vi "Beam deflector.vi"(6 "Sweep direction":bool, 7 "Level #":u8, 8 "Imbalance (V)":dbl min=-10.0 max=10.0 step=0.1 format="%.3f", 9 "Position (V)":dbl min=-10.0 max=10.0 step=0.1 format="%.3g", 10 "Angle (V)":dbl min=-10.0 max=10.0 step=0.1 format="%.3g", 11 "Focus (V)":dbl min=-10.0 max=10.0 step=0.1 format="%.3g") -> (3 "All posts":dbl[][](graph))   [LabVIEW 2018]
uses:
  <vilib>/Analysis/1siggen.llb/Ramp Pattern by Samples.vi
  <vilib>/Analysis/NI_AALBase.lvlib
panel:
  out "Post#1 down":dbl[](array[numeric])
  out "Post#1 up":dbl[](array[numeric])
  out "Post#2 up":dbl[](array[numeric])
  out "Post#2 down":dbl[](array[numeric])
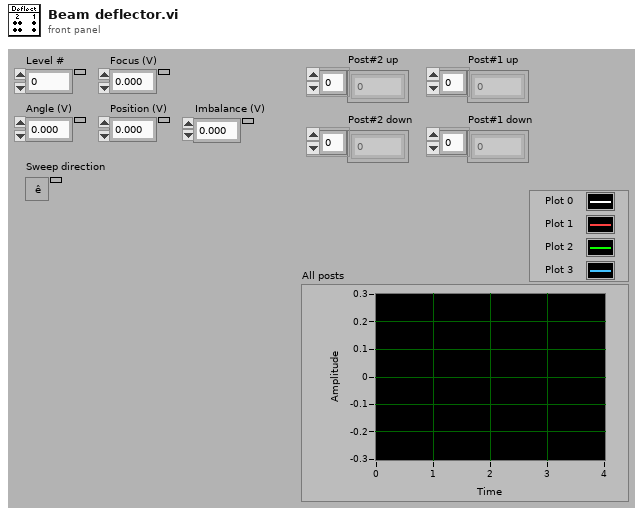
[diagram p1: front panel]
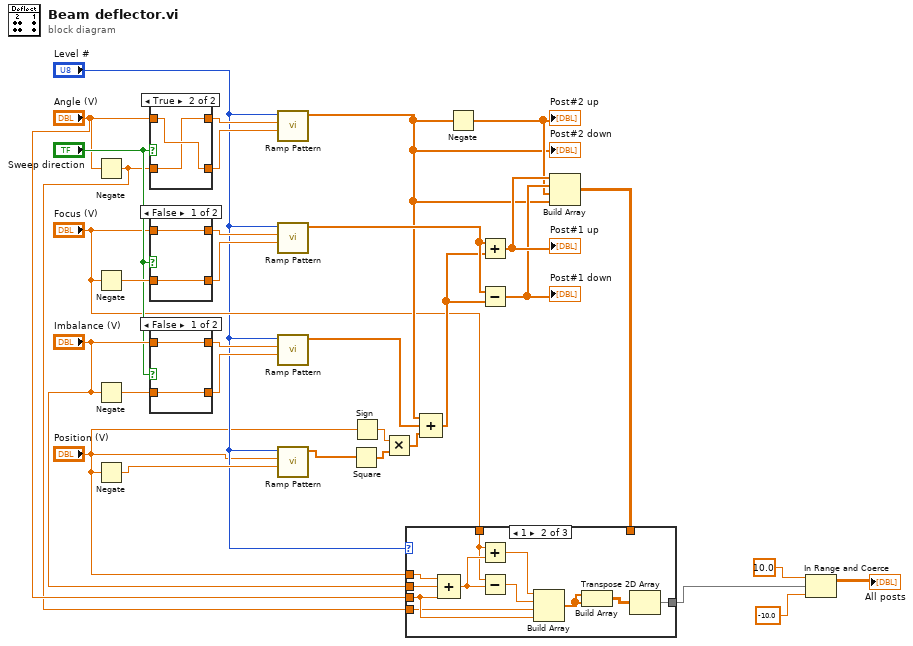
[diagram p0: block diagram]
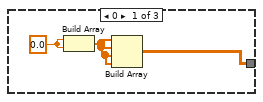
[diagram p2: hidden frame]
diagram:
  n1 = Negate(x="Angle (V)") -> (-x=w8:dbl)
  n2 = Negate(x="Focus (V)") -> (-x=w22:dbl)
  n3 = Negate(x="Imbalance (V)") -> (-x=w27:dbl)
  n4 = Negate(x="Position (V)") -> (-x=w25:dbl)
  n5 = case shown="True" "Sweep direction" {
    tunnel: "Angle (V)" -> [w34 w36]
    tunnel: [w34 w35] -> w24
    tunnel: w8 -> [w33 w35]
    tunnel: [w33 w36] -> w23
    frame False {
    }
    frame True {
    }
  }
  n6 = case shown="False" "Sweep direction" {
    tunnel: "Focus (V)" -> [w38 w40]
    tunnel: [w38 w39] -> w20
    tunnel: w22 -> [w37 w39]
    tunnel: [w37 w40] -> w19
    frame False {
    }
    frame True {
    }
  }
  n7 = case shown="False" "Sweep direction" {
    tunnel: "Imbalance (V)" -> [w42 w44]
    tunnel: [w42 w43] -> w29
    tunnel: w27 -> [w41 w43]
    tunnel: [w41 w44] -> w28
    frame False {
    }
    frame True {
    }
  }
  n8 = call-poly <vilib>:"Ramp Pattern.vi"("start"=w23, "end"=w24, "samples"="Level #") -> ("Ramp Pattern"=w11:dbl[])  [unwired: 7 in, 1 out]
  "Post#2 down" <- w11
  n9 = call-poly <vilib>:"Ramp Pattern.vi"("start"=w19, "end"=w20, "samples"="Level #") -> ("Ramp Pattern"=w16:dbl[])  [unwired: 7 in, 1 out]
  n10 = call-poly <vilib>:"Ramp Pattern.vi"("start"=w28, "end"=w29, "samples"="Level #") -> ("Ramp Pattern"=w17:dbl[])  [unwired: 7 in, 1 out]
  n11 = call-poly <vilib>:"Ramp Pattern.vi"("start"=w25, "end"="Position (V)", "samples"="Level #") -> ("Ramp Pattern"=w30:dbl[])  [unwired: 7 in, 1 out]
  n12 = Square(x=w30) -> (x^2=w32:dbl[])
  n13 = Sign(1:"Position (V)") -> (0:w31:dbl)
  n14 = Multiply(x=w31, y=w32) -> (x*y=w18:dbl[])
  n15 = Compound Arithmetic op=ADD(w11, w17, w18) -> (w15:dbl[])
  n16 = Negate(x=w11) -> (-x=w12:dbl[])
  "Post#2 up" <- w12
  n17 = Add(x=w16, y=w15) -> (x+y=w14:dbl[])
  "Post#1 up" <- w14
  n18 = Subtract(x=w16, y=w15) -> (x-y=w13:dbl[])
  "Post#1 down" <- w13
  n19 = Build Array(w14, w13, w12, w11) -> (w4:dbl[][])
  n20 = case shown="1" "Level #" {
    tunnel: "Imbalance (V)" -> [_ w58 _]
    tunnel: "Position (V)" -> [_ w57 _]
    tunnel: "Focus (V)" -> [_ w53 _]
    tunnel: "Angle (V)" -> [_ w52 _]
    tunnel: w8 -> [_ w51 _]
    tunnel: [w45 w48 w59] -> w3
    tunnel: w4 -> [_ _ w59]
    frame 0 {
      w47 = 0.0 ("element")
      n21 = Build Array(w47, w47) -> (w46:dbl[])
      n22 = Build Array(w46, w46, w46, w46) -> (w45:dbl[][])
    }
    frame 1 {
      n23 = Compound Arithmetic op=ADD(w57, w58, w52) -> (w56:dbl)
      n24 = Add(x=w53, y=w56) -> (x+y=w55:dbl)
      n25 = Subtract(x=w53, y=w56) -> (x-y=w54:dbl)
      n26 = Build Array(w55, w54, w51, w52) -> (w50:dbl[])
      n27 = Build Array(w50, w50) -> (w49:dbl[][])
      n28 = Transpose 2D Array(2D array=w49) -> (transposed array=w48:dbl[][])
    }
    frame Default {
    }
  }
  n29 = In Range and Coerce(upper limit=10.0 ("element"), x=w3, lower limit=-10.0 ("element")) -> (coerced(x)=→"All posts":dbl[][])  [unwired: 1 out]
